vi "Grid_Init.vi"(6 "Part of multigrid":bool, 7 "resume":T1, 8 "Error in":errorcluster, 9 "DC images in":dbl[][][](array[numeric]), 10 "Settings":T2={"Drift Correction Settings"={"Drift Correction every"=80, "Drift correction Pixels"=256, "Channel index (0-23)"=0, "MaxImagesBack"=2, "Threshold"=2, "Increment"=8, "max applied Drift Correction"=20, "Correct Drift"=TRUE, "Correlate"=0, "Correct z drift"=FALSE, "zdrift \nDuration (s)"=0.0}, "Spectroscopy Setting"={"Imaging Current"=1e-11, "ref Current"=7e-11, "tip Speed (m/s)"=2e-09, "Imaging Bias"=0.02, "ref Bias"=-0.1, "preSTS delay [ms]"=500, "STS z offset"=2e-10, "during Spec Bias (V)"=-0.1, "trigger1 < Hz"=0.0, "trigger 2 >Hz"=0.0, "autoStop"=FALSE, "Spectroscopy"=0, "PLL ON/OFF"=TRUE, "readjust setpoint every "=1, "z Reference"=FALSE, "Lock In"=TRUE}, "Misc"={"File name"="symmetric_node_zOff=200p", "Email when finished"="cornelius.krull@monash.edu,Dhaneesh.Gopalakrishnan@monash.edu,marina.castelli@monash.edu"}, "Grid Settings"={"type"=1, "type order"=1, "X pixel"=0, "Y pixel"=0, "Grid_Parms"={"center X (m)"=0.0, "center Y (m)"=0.0, "width (m)"=0.0, "height (m)"=0.0, "angle (deg)"=0.0}}} {"Grid Settings"."type order" items=["Line", "Grid"]; "Grid Settings"."type" items=["Line", "Grid"]; "Spectroscopy Setting"."Spectroscopy" items=["Bias", "zSpec"]; "Spectroscopy Setting"."trigger 2 >Hz" format="%#_6p"; "Spectroscopy Setting"."trigger1 < Hz" format="%#_6p"; "Spectroscopy Setting"."during Spec Bias (V)" format="%#_5p"; "Spectroscopy Setting"."STS z offset" format="%#_6p"; "Spectroscopy Setting"."ref Bias" format="%#_6p"; "Spectroscopy Setting"."Imaging Bias" format="%#_6p"; "Spectroscopy Setting"."tip Speed (m/s)" format="%.2p"; "Spectroscopy Setting"."ref Current" format="%#_6p"; "Spectroscopy Setting"."Imaging Current" format="%#_6p"; "Drift Correction Settings"."Correlate" items=["first Frame", "successive Frames"]; "Drift Correction Settings"."max applied Drift Correction" min=1 max=100 step=1 format="%.0p"; "Drift Correction Settings"."Threshold" min=1 step=1; "Drift Correction Settings"."Channel index (0-23)" items=["Current"=0, "Z (m)"=14]}, 11 "Application reference":refnum<vi>) -> (0 "error out":errorcluster, 1 "FileRefs":T3, 2 "Settings out":T2={"Drift Correction Settings"={"Drift Correction every"=80, "Drift correction Pixels"=256, "Channel index (0-23)"=0, "MaxImagesBack"=2, "Threshold"=2, "Increment"=8, "max applied Drift Correction"=20, "Correct Drift"=TRUE, "Correlate"=0, "Correct z drift"=FALSE, "zdrift \nDuration (s)"=0.0}, "Spectroscopy Setting"={"Imaging Current"=1e-11, "ref Current"=7e-11, "tip Speed (m/s)"=2e-09, "Imaging Bias"=0.02, "ref Bias"=-0.1, "preSTS delay [ms]"=500, "STS z offset"=2e-10, "during Spec Bias (V)"=-0.1, "trigger1 < Hz"=0.0, "trigger 2 >Hz"=0.0, "autoStop"=FALSE, "Spectroscopy"=0, "PLL ON/OFF"=TRUE, "readjust setpoint every "=1, "z Reference"=FALSE, "Lock In"=TRUE}, "Misc"={"File name"="symmetric_node_zOff=200p", "Email when finished"="cornelius.krull@monash.edu,Dhaneesh.Gopalakrishnan@monash.edu,marina.castelli@monash.edu"}, "Grid Settings"={"type"=1, "type order"=1, "X pixel"=0, "Y pixel"=0, "Grid_Parms"={"center X (m)"=0.0, "center Y (m)"=0.0, "width (m)"=0.0, "height (m)"=0.0, "angle (deg)"=0.0}}} caption="Settings" {"Grid Settings"."type order" items=["Line", "Grid"]; "Grid Settings"."type" items=["Line", "Grid"]; "Spectroscopy Setting"."Spectroscopy" items=["Bias", "zSpec"]; "Spectroscopy Setting"."trigger 2 >Hz" format="%#_6p"; "Spectroscopy Setting"."trigger1 < Hz" format="%#_6p"; "Spectroscopy Setting"."during Spec Bias (V)" format="%#_5p"; "Spectroscopy Setting"."STS z offset" format="%#_6p"; "Spectroscopy Setting"."ref Bias" format="%#_6p"; "Spectroscopy Setting"."Imaging Bias" format="%#_6p"; "Spectroscopy Setting"."tip Speed (m/s)" format="%.2p"; "Spectroscopy Setting"."ref Current" format="%#_6p"; "Spectroscopy Setting"."Imaging Current" format="%#_6p"; "Drift Correction Settings"."Correlate" items=["first Frame", "successive Frames"]; "Drift Correction Settings"."max applied Drift Correction" min=1 max=100 step=1 format="%.0p"; "Drift Correction Settings"."Threshold" min=1 step=1; "Drift Correction Settings"."Channel index (0-23)" items=["Current"=0, "Z (m)"=14]}, 3 "Application ref out":refnum<vi>, 5 "DC images out":dbl[][][](array[numeric]))   [LabVIEW 2021]
uses:
  <userlib>/Nanonis Prog Interface V5/Nanonis Prog Interface.lvlib
panel:
  # "RUN smart tilt before starting the GRID\nImg Angle = 0  CHECK CUTOFF\nmove tip to reference point for tip height"
  # "z Spectroscopy"
  # "GRID points"
  # "Increase this if no Drift was detected for \na certain number of images"
  # "% of image size"
  # "RUN smart tilt before starting the GRID\nImg Angle = 0  CHECK CUTOFF\nmove tip to reference point for tip height"
  # "z Spectroscopy"
  # "GRID points"
  # "Increase this if no Drift was detected for \na certain number of images"
  # "% of image size"
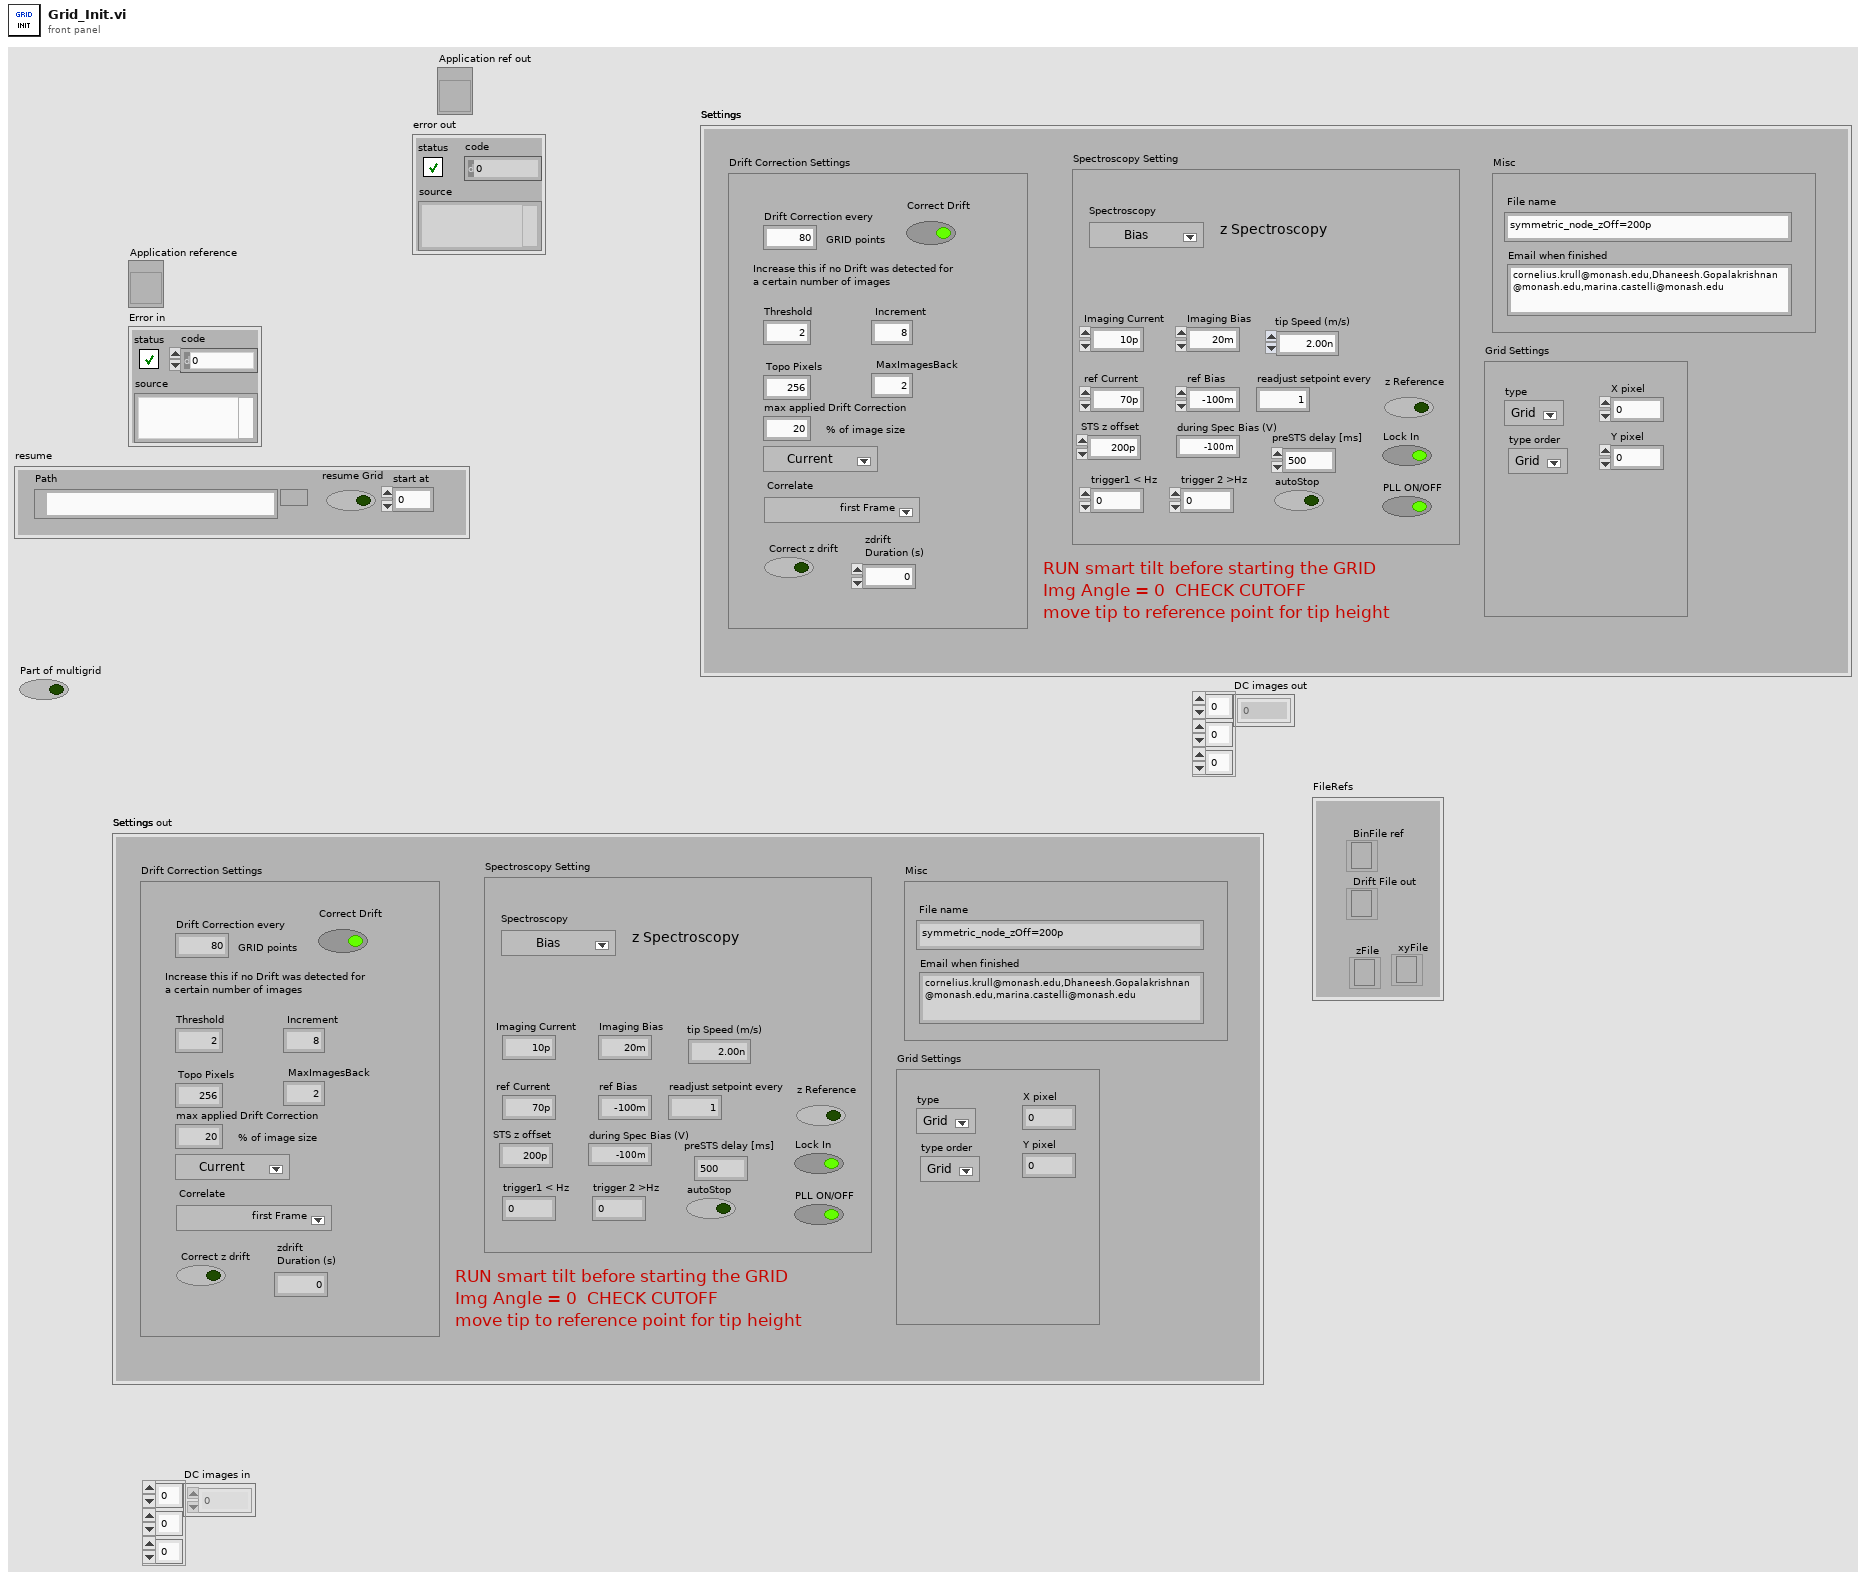
[diagram p1: front panel]
types:
  T1 = cluster{"resume Grid":bool, "Path":path, "start at":i32}
  T2 = cluster{"Drift Correction Settings":cluster{"Drift Correction every":i32, "Drift correction Pixels":i32, "Channel index (0-23)":u8, "MaxImagesBack":i32, "Threshold":i32, "Increment":i32, "max applied Drift Correction":i32, "Correct Drift":bool, "Correlate":u16, "Correct z drift":bool, "zdrift \nDuration (s)":dbl}, "Spectroscopy Setting":cluster{"Imaging Current":dbl, "ref Current":dbl, "tip Speed (m/s)":sgl, "Imaging Bias":dbl, "ref Bias":dbl, "preSTS delay [ms]":u32, "STS z offset":dbl, "during Spec Bias (V)":sgl, "trigger1 < Hz":sgl, "trigger 2 >Hz":sgl, "autoStop":bool, "Spectroscopy":u16, "PLL ON/OFF":bool, "readjust setpoint every ":i32, "z Reference":bool, "Lock In":bool}, "Misc":cluster{"File name":string, "Email when finished":string}, "Grid Settings":cluster{"type":u16, "type order":u16, "X pixel":i32, "Y pixel":i32, "Grid_Parms":cluster{"center X (m)":sgl, "center Y (m)":sgl, "width (m)":sgl, "height (m)":sgl, "angle (deg)":sgl}}}
  T3 = cluster{"Drift File out":refnum<file>, "zFile":refnum<file>, "BinFile ref":refnum<file>, "xyFile":refnum<file>}
  T4 = cluster{"type":u16, "type order":u16, "X pixel":i32, "Y pixel":i32, "Grid_Parms":cluster{"center X (m)":sgl, "center Y (m)":sgl, "width (m)":sgl, "height (m)":sgl, "angle (deg)":sgl}}
  T5 = cluster{"type":u16, "type order":u16, "X pixel":dbl, "Y pixel":dbl, "Grid_Parms":cluster{"center X (m)":sgl, "center Y (m)":sgl, "width (m)":sgl, "height (m)":sgl, "angle (deg)":sgl}}
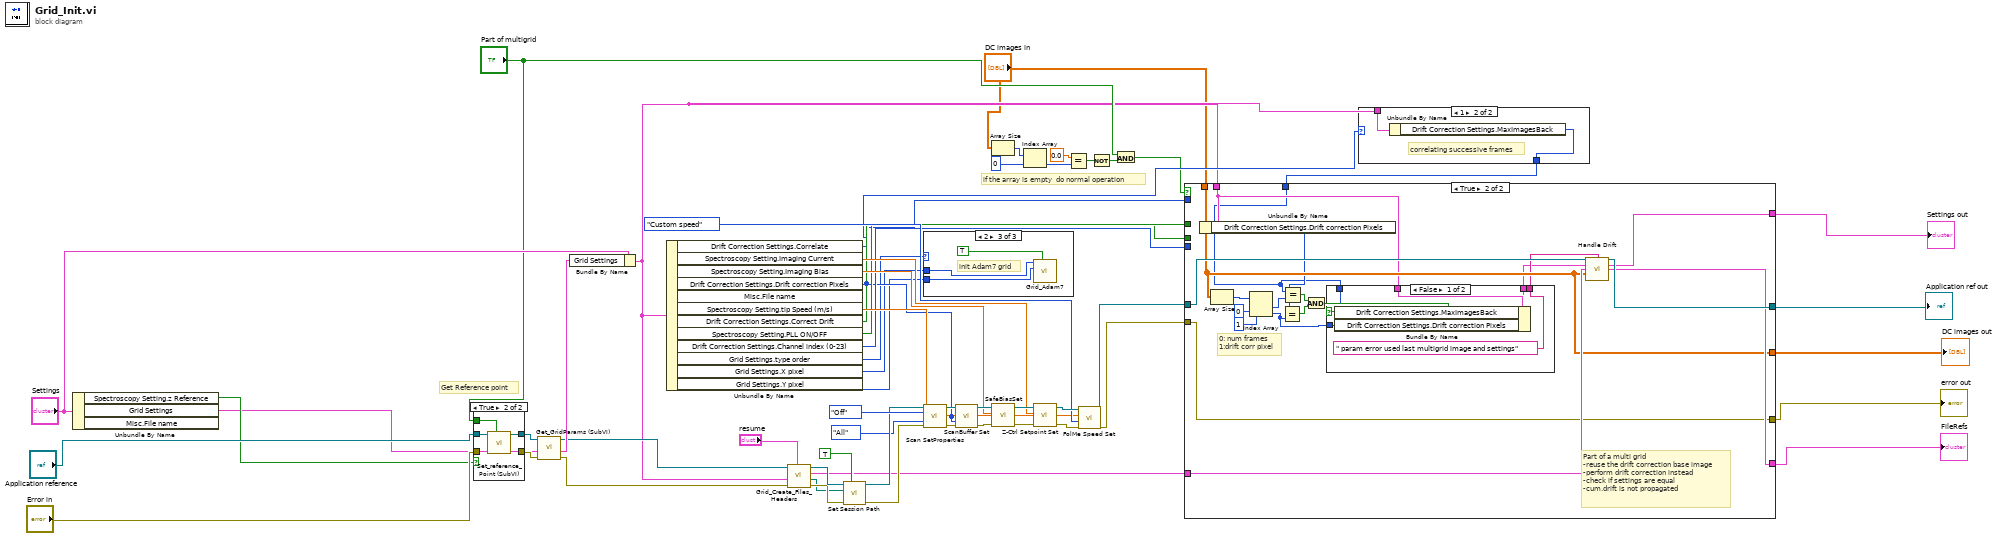
[diagram p0: block diagram]
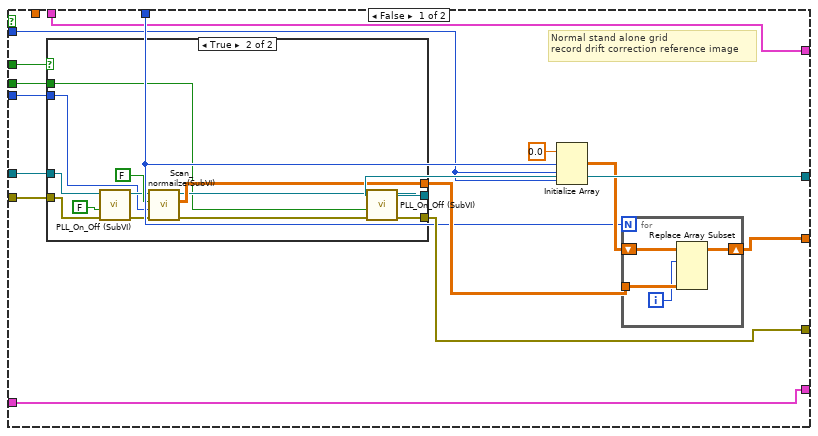
[diagram p2: hidden frame]
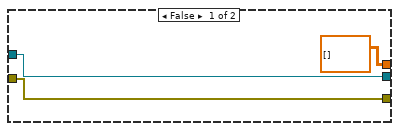
[diagram p3: hidden frame]
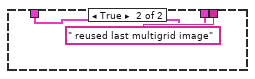
[diagram p4: hidden frame]
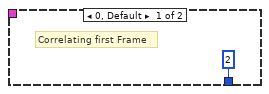
[diagram p7: hidden frame]
diagram:
  # "if the array is empty  do normal operation"
  # "Get Reference point"
  n1 = Unbundle By Name("Settings") -> ("Spectroscopy Setting.z Reference"=w56:bool, "Grid Settings"=w53:T4)  [unwired: 1 out]
  n2 = case shown="True" w56 {
    tunnel: "Application reference" -> [w60 w65]
    tunnel: "Error in" -> [w59 w64]
    tunnel: [w60 w63] -> w55
    tunnel: [w59 w62] -> w54
    tunnel: "Part of multigrid" -> [_ w61]
    frame False {
    }
    frame True {
      n3 = call "Set_reference_Point (SubVI).vi"("Part of multigrid"=w61, "error in (no error)"=w64, "Application in"=w65) -> ("error out"=w62:errorcluster, "Application out"=w63:refnum<vi>)  [unwired: 7 in]
    }
  }
  n4 = call "Get_GridParams (SubVI).vi"("error in (no error)"=w54, "Grid Settings"=w53, "Application in"=w55) -> ("error out"=w49:errorcluster, "Grid Settings"=w51:T5, "Application out"=w50:refnum<vi>)  [unwired: 5 in, 1 out]
  n5 = Bundle By Name(cluster="Settings", "Grid Settings"=w51) -> (w12:T2)
  n6 = Unbundle By Name(w12) -> ("Drift Correction Settings.Correlate"=w18:u16, "Spectroscopy Setting.Imaging Current"=w34:dbl, "Spectroscopy Setting.Imaging Bias"=w37:dbl, "Drift Correction Settings.Drift correction Pixels"=w19:i32, "Spectroscopy Setting.tip Speed (m/s)"=w30:sgl, "Drift Correction Settings.Correct Drift"=w25:bool, "Spectroscopy Setting.PLL ON/OFF"=w24:bool, "Drift Correction Settings.Channel index (0-23)"=w23:u8, "Grid Settings.type order"=w17:u16, "Grid Settings.X pixel"=w16:i32, "Grid Settings.Y pixel"=w15:i32)  [unwired: 1 out]
  n7 = call "Grid_Create_Files_Headers.vi"("resume"="resume", "Error in (no error)"=w49, "Settings"=w12, "Application ref in"=w50) -> ("error out"=w46:errorcluster, "topoFilePath"=w22:path, "FileRefs"=w10:T3, "Application ref out"=w48:refnum<vi>)  [unwired: 4 in]
  n8 = call <userlib>:"Set Session Path.vi"("Save settings to previous? (False)"=TRUE, "error in (no error)"=w46, "Session Folder"=w22, "Application ref in"=w48) -> ("error out"=w41:errorcluster, "Application ref out"=w42:refnum<vi>)  [unwired: 6 in]
  n9 = case shown="2" w17 {
    tunnel: w16 -> [_ _ w67]
    tunnel: w15 -> [_ _ w66]
    frame 0, Default {
    }
    frame 1 {
    }
    frame 2 {
      # "init Adam7 grid"
      n10 = call "Grid_Adam7.vi"("reset"=TRUE, "py 2"=w66, "px 2"=w67) -> ()  [unwired: 7 in, 2 out]
    }
  }
  n11 = call <userlib>:"Scan SetProperties.vi"("Application ref in"=w42, "Continuous scan"=enum16{"No change", "On", "Off"}."Off", "Auto save"=enum16{"No change", "All", "Next", "Off"}."All", "Error in (no error)"=w41) -> ("Application ref out"=w44:refnum<vi>, "Error out"=w43:errorcluster)  [unwired: 10 in]
  n12 = call <userlib>:"ScanBuffer Set.vi"("Application ref in"=w44, "Pixels"=w19, "Lines"=w19, "error in (no error)"=w43) -> ("Application ref out"=w39:refnum<vi>, "error out"=w38:errorcluster)  [unwired: 10 in]
  n13 = Array Size(array="DC images in") -> (size(s)=w6:i32[])
  n14 = call "SafeBiasSet.vi"("Application ref in"=w39, "Bias (V)"=w37, "error in (no error)"=w38) -> ("Application ref out"=w35:refnum<vi>, "Error out"=w36:errorcluster)  [unwired: 6 in]
  n15 = Index Array(array=w6, index=0) -> (element=w2:i32)
  n16 = call <userlib>:"Z-Ctrl Setpoint Set.vi"("error in (no error)"=w36, "Z Controller setpoint"=w34, "Application ref in"=w35) -> ("error out"=w32:errorcluster, "Application ref out"=w33:refnum<vi>)  [unwired: 7 in]
  n17 = Equal?(x=0.0, y=w2) -> (x = y?=w3:bool)
  n18 = call <userlib>:"FolMe Speed Set.vi"("error in (no error)"=w32, "Speed Setting (Custom)"=enum32{"Scan speed", "Custom speed"}."Custom speed", "Speed (m/s)"=w30, "Application ref in"=w33) -> ("error out"=w28:errorcluster, "Application ref out"=w29:refnum<vi>)  [unwired: 4 in]
  n19 = Not(x=w3) -> (.not. x?=w1:bool)
  n20 = And(x="Part of multigrid", y=w1) -> (x .and. y?=w8:bool)
  n21 = case shown="1" w18 {
    tunnel: w12 -> [_ w71]
    tunnel: [2 ("MaxImagesBack") w70] -> w21
    frame 0, Default {
      # "Correlating first Frame"
    }
    frame 1 {
      # "correlating successive frames"
      n22 = Unbundle By Name(w71) -> ("Drift Correction Settings.MaxImagesBack"=w70:i32)
    }
  }
  n23 = case shown="True" w8 {
    tunnel: w29 -> [w86 w126]
    tunnel: w28 -> [w85 w107]
    tunnel: [w84 w107] -> w27
    tunnel: [w83 w125] -> w26
    tunnel: w25 -> [w82 _]
    tunnel: w24 -> [w81 _]
    tunnel: w23 -> [w80 _]
    tunnel: w21 -> [w76 w110]
    tunnel: [w75 w121] -> w20
    tunnel: w19 -> [w74 _]
    tunnel: w12 -> [w73 w111]
    tunnel: [w73 w124] -> w11
    tunnel: w10 -> [w72 w123]
    tunnel: [w72 w122] -> w9
    tunnel: "DC images in" -> [_ w121]
    frame False {
      # "Normal stand alone grid\nrecord drift correction reference image"
      n24 = case shown="True" w82 {
        tunnel: [dbl[][] [] ("Array") w106] -> w77
        tunnel: w86 -> [w93 w104]
        tunnel: [w93 w100] -> w83
        tunnel: w85 -> [w91 w99]
        tunnel: [w91 w96] -> w84
        tunnel: w81 -> [_ w95]
        tunnel: w80 -> [_ w94]
        frame False {
        }
        frame True {
          n25 = call "PLL_On_Off (SubVI).vi"("error in (no error)"=w99, "Output ON/OFF (F=OFF)"=FALSE, "Application in"=w104) -> ("error out"=w98:errorcluster, "Application out"=w103:refnum<vi>)  [unwired: 7 in]
          n26 = call "Scan_normailze(SubVI).vi"("error in (no error)"=w98, "Channel index (0-23)"=w94, "Normalization"=FALSE ("Boolean"), "Application in"=w103) -> ("error out"=w97:errorcluster, "Array"=w106:dbl[][], "Application out"=w101:refnum<vi>)  [unwired: 5 in]
          n27 = call "PLL_On_Off (SubVI).vi"("error in (no error)"=w97, "Output ON/OFF (F=OFF)"=w95, "Application in"=w101) -> ("error out"=w96:errorcluster, "Application out"=w100:refnum<vi>)  [unwired: 7 in]
        }
      }
      n28 = Initialize Array(0.0 ("element"), w76, w74, w74) -> (w78:dbl[][][])
      n29 = for {
        N: w76 -> [_]
        tunnel: w77 -> [w89]
        shift-right: [w88] -> w75
        shift-left: w78 -> [w90]
        i -> [w87]
        n30 = Replace Array Subset(array=w90, new element=w89, index (dim 0)=w87) -> (w88:dbl[][][])  [unwired: 2 in]
      }
    }
    frame True {
      # "0: num frames\n1:drift corr pixel"
      # "Part of a multi grid\n-reuse the drift correction base image\n-perform drift correction instead\n-check if settings are equal\n-cum.drift is not propagated"
      n31 = Unbundle By Name(w111) -> ("Drift Correction Settings.Drift correction Pixels"=w116:i32)
      n32 = Array Size(array=w121) -> (size(s)=w120:i32[])
      n33 = Index Array(array=w120, index #1=0 ("index"), index #2=1 ("index")) -> (element #1=w117:i32, element #2=w108:i32)
      n34 = Equal?(x=w116, y=w108) -> (x = y?=w114:bool)
      n35 = Equal?(x=w110, y=w117) -> (x = y?=w115:bool)
      n36 = And(x=w115, y=w114) -> (x .and. y?=w113:bool)
      n37 = case shown="False" w113 {
        tunnel: [" param error used last multigrid image and settings" ("Add.comment") " reused last multigrid image" ("Add.comment")] -> w112
        tunnel: w111 -> [w130 w132]
        tunnel: w110 -> [w129 _]
        tunnel: [w128 w132] -> w109
        tunnel: w108 -> [w127 _]
        frame False {
          n38 = Bundle By Name(cluster=w130, "Drift Correction Settings.MaxImagesBack"=w129, "Drift Correction Settings.Drift correction Pixels"=w127) -> (w128:T2)
        }
        frame True {
        }
      }
      n39 = call "Handle Drift.vi"("Application ref in"=w126, "Add.comment"=w112, "Settings"=w109, "FileRefs"=w123, "Drift Correction image"=w121) -> ("Application out"=w125:refnum<vi>, "Settings out"=w124:T2, "FileRefs out File Refs  Out"=w122:T3)  [unwired: 5 in, 3 out]
    }
  }
  "Application ref out" <- w26
  "error out" <- w27
  "FileRefs" <- w9
  "DC images out" <- w20
  "Settings out" <- w11
